vi "Service Location FGV.vi"(8 "error in":errorcluster, 10 "Resolve Service Request":T1, 11 "Action":enum16{"Get Service Location", "Clear Cache"}(ring)) -> (0 "error out":errorcluster, 3 "Service Location":T2)   [LabVIEW 2020, in "MeasurementLink Measurement Server.lvlib"]
uses:
  MeasurementLink Measurement Server.lvlib
  MeasurementLink Discovery Client/RPC Messages/ni_measurementlink_discovery_v1_ServiceLocation.ctl
  MeasurementLink Discovery Client/RPC Messages/ni_measurementlink_discovery_v1_ResolveServiceRequest.ctl
  FGV Action.ctl
  MeasurementLink Discovery Client/MeasurementLink Discovery Client.lvlib
  GrpcClientPool.lvclass
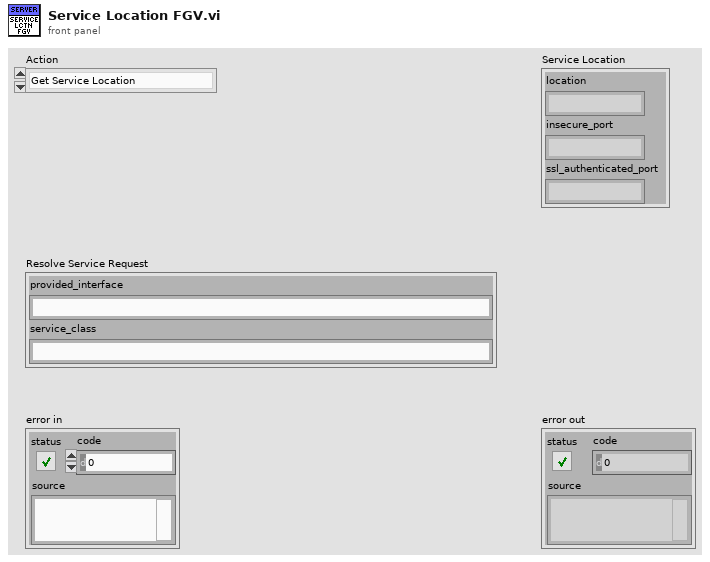
[diagram p1: front panel]
types:
  T1 = typedef "MeasurementLink Discovery Client.lvlib/ni_measurementlink_discovery_v1_ResolveServiceRequest.ctl" = cluster{"provided_interface":string, "service_class":string}
  T2 = typedef "MeasurementLink Discovery Client.lvlib/ni_measurementlink_discovery_v1_ServiceLocation.ctl" = cluster{"location":string, "insecure_port":string, "ssl_authenticated_port":string}
  T3 = typedef "MeasurementLink Measurement Server.lvlib/GrpcClientPool.lvclass/FGV Action.ctl" = enum16{"Get Discovery Client", "Get Session Client", "Get Pinmap Client", "Destroy Clients"}
  T4 = typedef "grpc-lvsupport-release.lvlib/grpcId.ctl" = u64
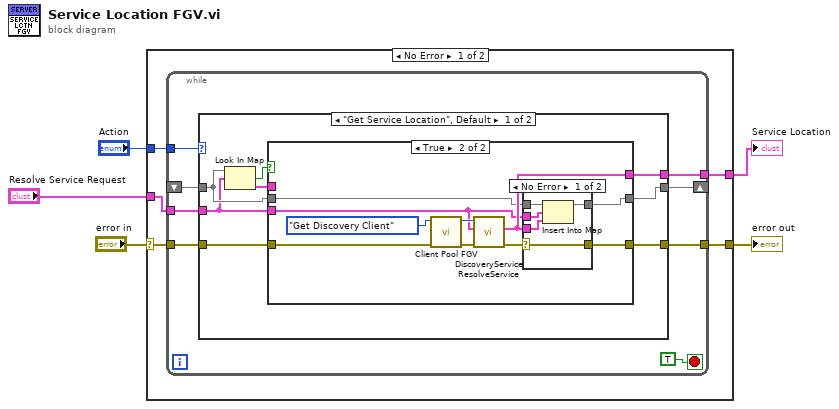
[diagram p0: block diagram]
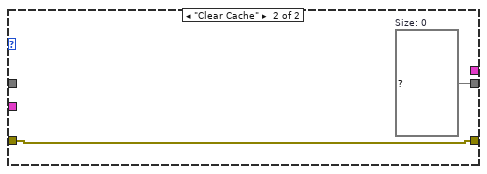
[diagram p4: hidden frame]
diagram:
  n1 = case shown="No Error" "error in" {
    selector: "error in" -> [w10 w49]
    tunnel: [w7 w49] -> w2
    tunnel: [w9 _] -> w5
    tunnel: "Resolve Service Request" -> [w8 _]
    tunnel: "Action" -> [w6 _]
    frame No Error {
      n2 = while {
        shift-right: [w13] -> _
        shift-left: _ -> [w16]
        tunnel: w10 -> [w17]
        tunnel: [w15] -> w9
        tunnel: w8 -> [w14]
        tunnel: [w12] -> w7
        tunnel: w6 -> [w11]
        stop <- TRUE stop-if-true
        n3 = case shown="\"Get Service Location\", Default" w11 {
          tunnel: w16 -> [w25 _]
          tunnel: [w23 _] -> w15
          tunnel: w14 -> [w22 _]
          tunnel: w17 -> [w21 w47]
          tunnel: [w20 w48] -> w13
          tunnel: [w19 w47] -> w12
          frame "Get Service Location", Default {
            n4 = Look In Map(map=w25, key=w22) -> (key not found?=w26:bool, value=w24:T2)  [unwired: 1 in]
            n5 = case shown="True" w26 {
              tunnel: w25 -> [w28 w34]
              tunnel: w24 -> [w29 _]
              tunnel: [w29 w35] -> w23
              tunnel: w22 -> [_ w33]
              tunnel: w21 -> [w27 w38]
              tunnel: [w28 w32] -> w20
              tunnel: [w27 w30] -> w19
              frame False {
              }
              frame True {
                n6 = call "Client Pool FGV.vi"("error in (no error)"=w38, "Action"=FGV_Action."Get Discovery Client") -> ("error out"=w37:errorcluster, "grpc client id"=w36:T4)  [unwired: 8 in]
                n7 = call "DiscoveryService ResolveService.vi"("error in"=w37, "Request Data"=w33, "gRPC ID"=w36) -> ("error out"=w31:errorcluster, "Response Data"=w35:T2)  [unwired: 6 in, 1 out]
                n8 = case shown="No Error" w31 {
                  selector: w31 -> [w40 w46]
                  tunnel: w35 -> [w44 _]
                  tunnel: w34 -> [w43 w45]
                  tunnel: w33 -> [w42 _]
                  tunnel: [w41 w45] -> w32
                  tunnel: [w40 w46] -> w30
                  frame No Error {
                    n9 = Insert Into Map(map in=w43, key=w42, value=w44) -> (map out=w41:map{T1, T2})  [unwired: 2 out]
                  }
                  frame Error {
                  }
                }
              }
            }
          }
          frame "Clear Cache" {
            w48 = map{T1, T2} {}  # Size: 0
          }
        }
      }
    }
    frame Error {
    }
  }
  "Service Location" <- w5
  "error out" <- w2
